vi "Parse Sentence_GGA.vi"(8 "error in (no error)":errorcluster, 11 "GGA sentence":string) -> (0 "error out":errorcluster, 3 "GGA_Data":T1 {"fix quality"."quality" items=["Invalid", "GPS Fix", "DGPS Fix", "PPS Fix", "Real Time Kinematic", "Float RTK", "Estimated", "Manual Input Mode", "Simulation Mode"]})   [LabVIEW 2024]
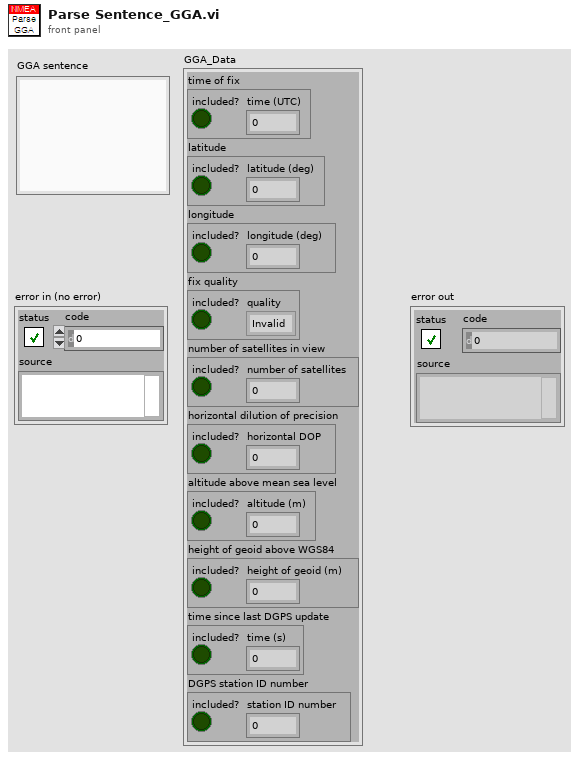
[diagram p1: front panel]
types:
  T1 = cluster{"time of fix":cluster{"included?":bool, "time (UTC)":dbl}, "latitude":cluster{"included?":bool, "latitude (deg)":dbl}, "longitude":cluster{"included?":bool, "longitude (deg)":dbl}, "fix quality":cluster{"included?":bool, "quality":u16}, "number of satellites in view":cluster{"included?":bool, "number of satellites":i8}, "horizontal dilution of precision":cluster{"included?":bool, "horizontal DOP":dbl}, "altitude above mean sea level":cluster{"included?":bool, "altitude (m)":dbl}, "height of geoid above WGS84":cluster{"included?":bool, "height of geoid (m)":dbl}, "time since last DGPS update":cluster{"included?":bool, "time (s)":dbl}, "DGPS station ID number":cluster{"included?":bool, "station ID number":dbl}}
  T2 = cluster{"Valid?":bool, "Number of Satellites":i8}
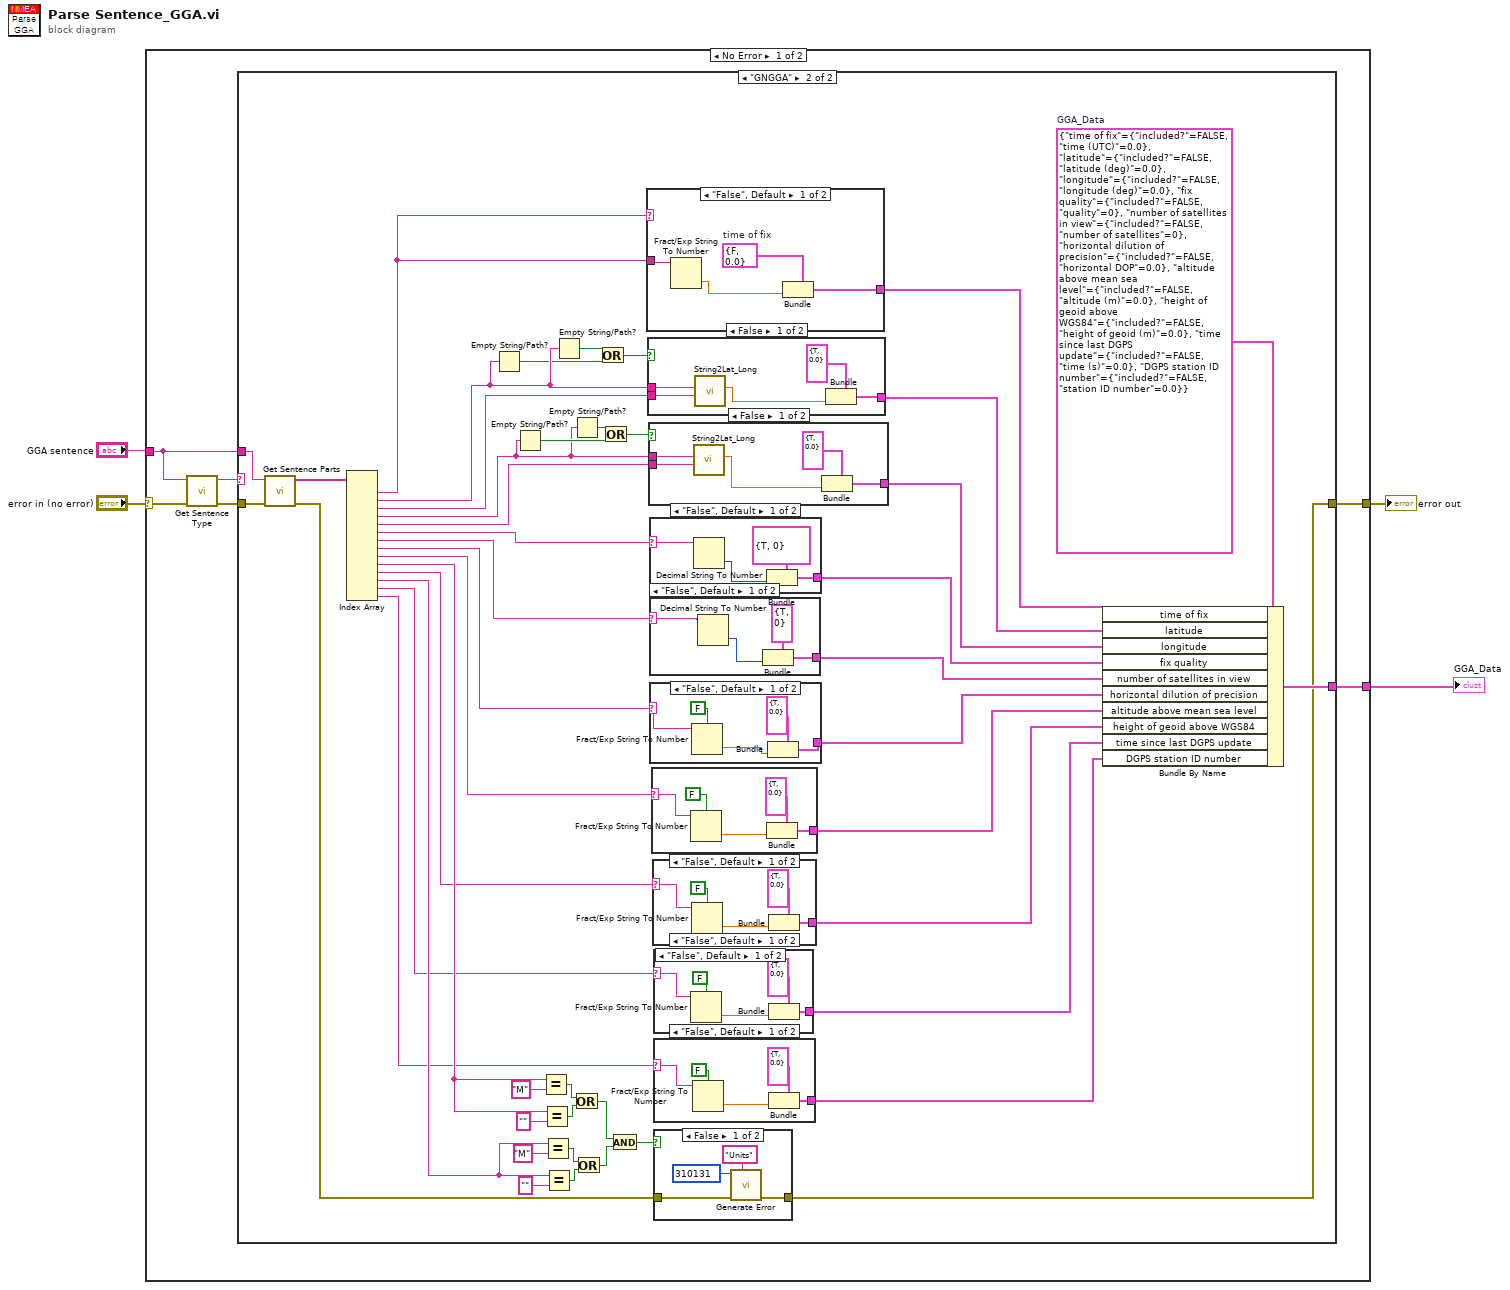
[diagram p0: block diagram]
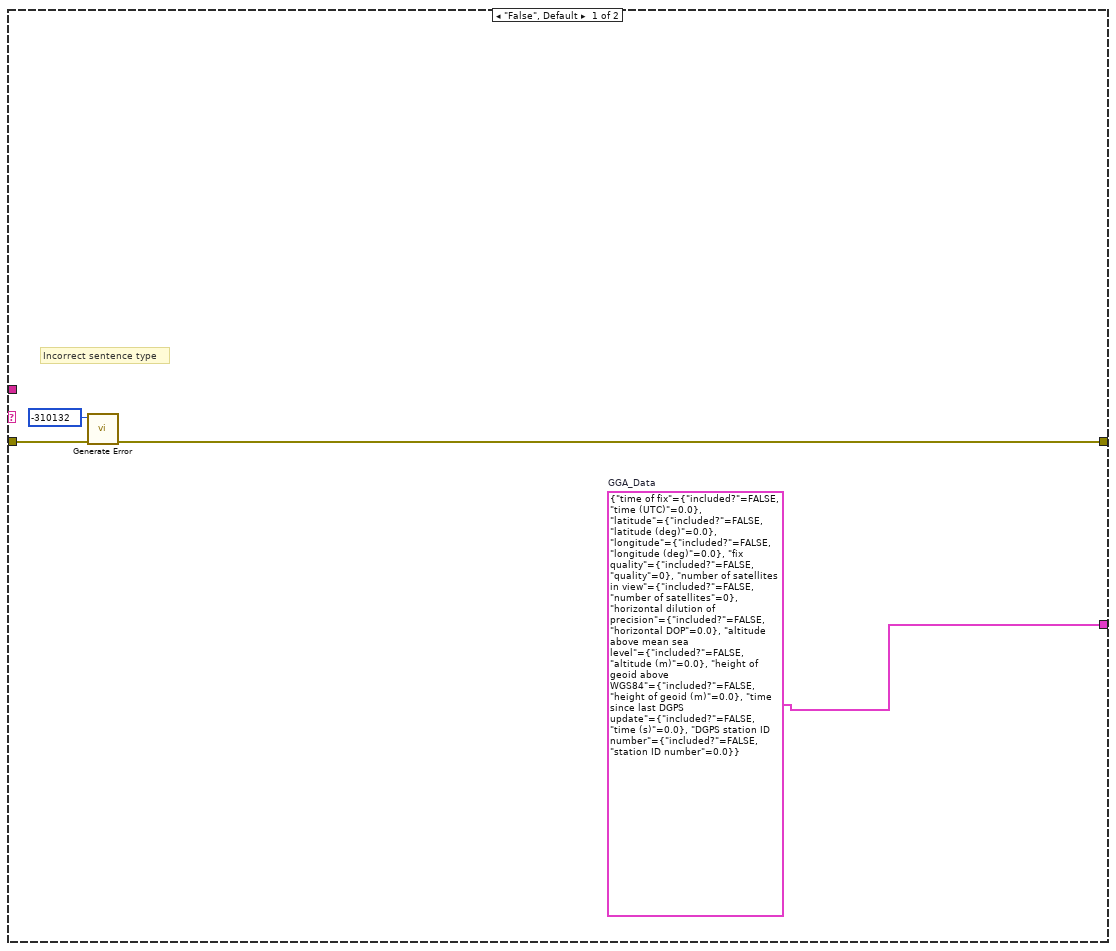
[diagram p2: hidden frame]
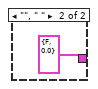
[diagram p4: hidden frame]
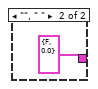
[diagram p5: hidden frame]
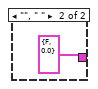
[diagram p6: hidden frame]
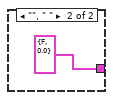
[diagram p7: hidden frame]
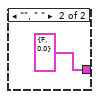
[diagram p8: hidden frame]
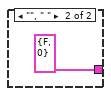
[diagram p9: hidden frame]
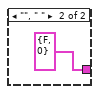
[diagram p10: hidden frame]
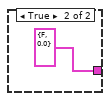
[diagram p11: hidden frame]
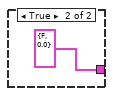
[diagram p12: hidden frame]
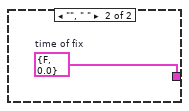
[diagram p13: hidden frame]
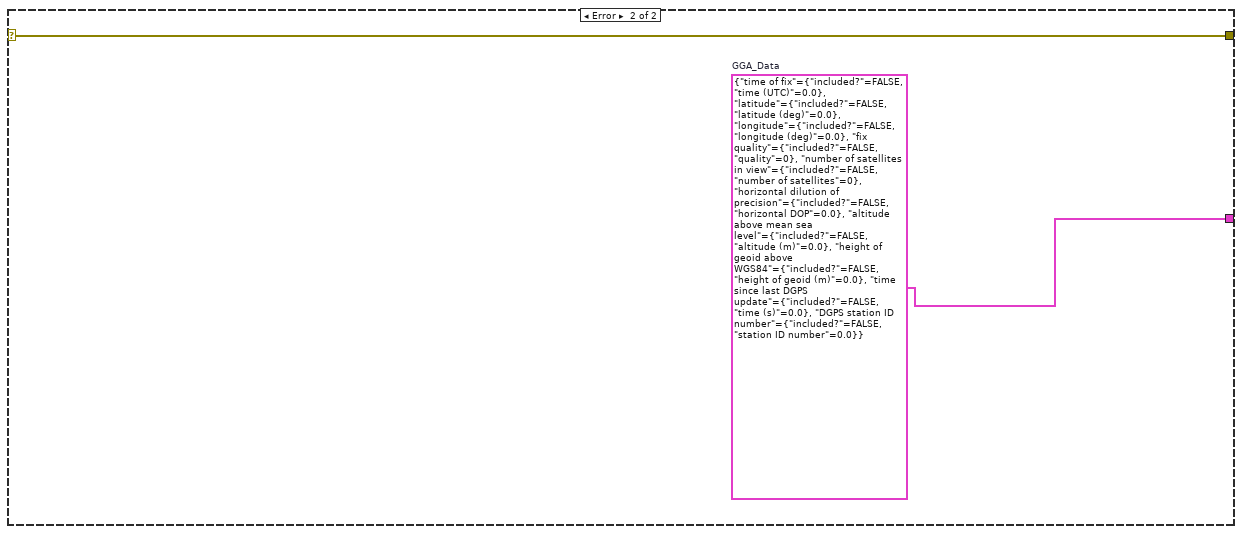
[diagram p14: hidden frame]
diagram:
  n1 = case shown="No Error" "error in (no error)" {
    selector: "error in (no error)" -> [w8 w126]
    tunnel: [w9 w126] -> w2
    tunnel: [w10 w125] -> w1
    tunnel: "GGA sentence" -> [w6 _]
    frame No Error {
      n2 = call "Get Sentence Type.vi"("error in (no error)"=w8, "sentence"=w6) -> ("error out"=w7:errorcluster, "sentence type"=w5:string)  [unwired: 7 in, 1 out]
      n3 = case shown="\"GNGGA\"" w5 {
        tunnel: [w11 w62] -> w10
        tunnel: w6 -> [_ w18]
        tunnel: w7 -> [w13 w61]
        tunnel: [w12 w42] -> w9
        frame "False", Default {
          w11 = T1 {"time of fix"={"included?"=FALSE, "time (UTC)"=0.0}, "latitude"={"included?"=FALSE, "latitude (deg)"=0.0}, "longitude"={"included?"=FALSE, "longitude (deg)"=0.0}, "fix quality"={"included?"=FALSE, "quality"=0}, "number of satellites in view"={"included?"=FALSE, "number of satellites"=0}, "horizontal dilution of precision"={"included?"=FALSE, "horizontal DOP"=0.0}, "altitude above mean sea level"={"included?"=FALSE, "altitude (m)"=0.0}, "height of geoid above WGS84"={"included?"=FALSE, "height of geoid (m)"=0.0}, "time since last DGPS update"={"included?"=FALSE, "time (s)"=0.0}, "DGPS station ID number"={"included?"=FALSE, "station ID number"=0.0}}  # GGA_Data
          # "Incorrect sentence type"
          n4 = call "Generate Error.vi"("error in (no error)"=w13, "code"=-310132) -> ("error out"=w12:errorcluster)  [unwired: 9 in]
        }
        frame "GNGGA" {
          w16 = T1 {"time of fix"={"included?"=FALSE, "time (UTC)"=0.0}, "latitude"={"included?"=FALSE, "latitude (deg)"=0.0}, "longitude"={"included?"=FALSE, "longitude (deg)"=0.0}, "fix quality"={"included?"=FALSE, "quality"=0}, "number of satellites in view"={"included?"=FALSE, "number of satellites"=0}, "horizontal dilution of precision"={"included?"=FALSE, "horizontal DOP"=0.0}, "altitude above mean sea level"={"included?"=FALSE, "altitude (m)"=0.0}, "height of geoid above WGS84"={"included?"=FALSE, "height of geoid (m)"=0.0}, "time since last DGPS update"={"included?"=FALSE, "time (s)"=0.0}, "DGPS station ID number"={"included?"=FALSE, "station ID number"=0.0}}  # GGA_Data
          n5 = call "Get Sentence Parts.vi"("error in (no error)"=w61, "sentence"=w18) -> ("error out"=w46:errorcluster, "sentence data"=w17:string[])  [unwired: 7 in, 1 out]
          n6 = Index Array(array=w17) -> (element #1=w26:string, element #2=w56:string, element #3=w60:string, element #4=w52:string, element #5=w59:string, element #6=w25:string, element #7=w24:string, element #8=w23:string, element #9=w22:string, element #10=w41:string, element #11=w21:string, element #12=w35:string, element #13=w20:string, element #14=w19:string)  [unwired: 14 in]
          n7 = Empty String/Path?(string/path=w56) -> (empty?=w55:bool)
          n8 = Empty String/Path?(string/path=w52) -> (empty?=w54:bool)
          n9 = Equal?(x=w41, y="M") -> (x = y?=w44:bool)
          n10 = Equal?(x=w41, y="") -> (x = y?=w45:bool)
          n11 = Equal?(x=w35, y="M") -> (x = y?=w37:bool)
          n12 = Equal?(x=w35, y="") -> (x = y?=w36:bool)
          n13 = Empty String/Path?(string/path=w56) -> (empty?=w57:bool)
          n14 = Empty String/Path?(string/path=w52) -> (empty?=w53:bool)
          n15 = Or(x=w44, y=w45) -> (x .or. y?=w33:bool)
          n16 = Or(x=w37, y=w36) -> (x .or. y?=w32:bool)
          n17 = Or(x=w57, y=w55) -> (x .or. y?=w58:bool)
          n18 = Or(x=w53, y=w54) -> (x .or. y?=w51:bool)
          n19 = And(x=w33, y=w32) -> (x .and. y?=w34:bool)
          n20 = case shown="\"False\", Default" w26 {
            tunnel: [w123 w124] -> w15
            tunnel: w26 -> [w121 _]
            frame "False", Default {
              w122 = cluster{"included?":bool, "time (UTC)":dbl} {"included?"=FALSE, "time (UTC)"=0.0}  # time of fix
              n21 = Fract/Exp String To Number(string=w121) -> (number=w120:dbl)  [unwired: 4 out]
              n22 = Bundle(cluster=w122, "time (UTC)"=w120) -> (w123:cluster{"included?":bool, "time (UTC)":dbl})  [unwired: 1 out]
            }
            frame "", " " {
              w124 = cluster{"included?":bool, "time (UTC)":dbl} {"included?"=FALSE, "time (UTC)"=0.0}  # time of fix
            }
          }
          n23 = case shown="False" w58 {
            tunnel: [w116 cluster{"Valid?":bool, "Latitude (Deg)":dbl} {"Valid?"=FALSE, "Latitude (Deg)"=0.0} ("Latitude")] -> w48
            tunnel: w56 -> [w118 _]
            tunnel: w60 -> [w117 _]
            frame False {
              n24 = call "String2Lat_Long.vi"("direction string"=w117, "numeric string for lat/lon"=w118) -> ("composite value"=w114:dbl)  [unwired: 9 in]
              n25 = Bundle(cluster=cluster{"Valid?":bool, "Latitude (Deg)":dbl} {"Valid?"=TRUE, "Latitude (Deg)"=0.0} ("Latitude"), "Latitude (Deg)"=w114) -> (w116:cluster{"Valid?":bool, "Latitude (Deg)":dbl})  [unwired: 1 out]
            }
            frame True {
            }
          }
          n26 = case shown="False" w51 {
            tunnel: w59 -> [w112 _]
            tunnel: w52 -> [w111 _]
            tunnel: [w108 cluster{"Valid?":bool, "Longitude (Deg)":dbl} {"Valid?"=FALSE, "Longitude (Deg)"=0.0} ("Longitude")] -> w47
            frame False {
              n27 = call "String2Lat_Long.vi"("direction string"=w112, "numeric string for lat/lon"=w111) -> ("composite value"=w110:dbl)  [unwired: 9 in]
              n28 = Bundle(cluster=cluster{"Valid?":bool, "Longitude (Deg)":dbl} {"Valid?"=TRUE, "Longitude (Deg)"=0.0} ("Longitude"), "Longitude (Deg)"=w110) -> (w108:cluster{"Valid?":bool, "Longitude (Deg)":dbl})  [unwired: 1 out]
            }
            frame True {
            }
          }
          n29 = case shown="\"False\", Default" w25 {
            selector: w25 -> [w103 _]
            tunnel: [w104 cluster{"Valid?":bool, "Fix Quality":u16} {"Valid?"=FALSE, "Fix Quality"=0} ("Fix Quality")] -> w50
            frame "False", Default {
              n30 = Decimal String To Number(string=w103) -> (number=w105:i32)  [unwired: 3 out]
              n31 = Bundle(cluster=cluster{"Valid?":bool, "Fix Quality":u16} {"Valid?"=TRUE, "Fix Quality"=0} ("Fix Quality"), "Fix Quality"=w105) -> (w104:cluster{"Valid?":bool, "Fix Quality":u16})  [unwired: 1 out]
            }
            frame "", " " {
            }
          }
          n32 = case shown="\"False\", Default" w24 {
            selector: w24 -> [w98 _]
            tunnel: [w99 T2 {"Valid?"=FALSE, "Number of Satellites"=0} ("Number of Satellites Being Tracked")] -> w49
            frame "False", Default {
              n33 = Decimal String To Number(string=w98) -> (number=w101:i32)  [unwired: 3 out]
              n34 = Bundle(cluster=T2 {"Valid?"=TRUE, "Number of Satellites"=0} ("Number of Satellites Being Tracked"), "Number of Satellites"=w101) -> (w99:T2)  [unwired: 1 out]
            }
            frame "", " " {
            }
          }
          n35 = case shown="\"False\", Default" w23 {
            selector: w23 -> [w93 _]
            tunnel: [w94 cluster{"Valid?":bool, "Horizontal DOP":dbl} {"Valid?"=FALSE, "Horizontal DOP"=0.0} ("Horizontal Dilution of Precision")] -> w31
            frame "False", Default {
              n36 = Fract/Exp String To Number(use system decimal point (T)=FALSE, string=w93) -> (number=w95:dbl)  [unwired: 3 out]
              n37 = Bundle(cluster=cluster{"Valid?":bool, "Horizontal DOP":dbl} {"Valid?"=TRUE, "Horizontal DOP"=0.0} ("Horizontal Dilution of Precision"), "Horizontal DOP"=w95) -> (w94:cluster{"Valid?":bool, "Horizontal DOP":dbl})  [unwired: 1 out]
            }
            frame "", " " {
            }
          }
          n38 = case shown="\"False\", Default" w22 {
            selector: w22 -> [w87 _]
            tunnel: [w88 cluster{"Valid?":bool, "Horizontal DOP":dbl} {"Valid?"=FALSE, "Horizontal DOP"=0.0} ("Horizontal Dilution of Precision")] -> w30
            frame "False", Default {
              n39 = Fract/Exp String To Number(use system decimal point (T)=FALSE, string=w87) -> (number=w89:dbl)  [unwired: 3 out]
              n40 = Bundle(cluster=cluster{"Valid?":bool, "Horizontal DOP":dbl} {"Valid?"=TRUE, "Horizontal DOP"=0.0} ("Horizontal Dilution of Precision"), "Horizontal DOP"=w89) -> (w88:cluster{"Valid?":bool, "Horizontal DOP":dbl})  [unwired: 1 out]
            }
            frame "", " " {
            }
          }
          n41 = case shown="\"False\", Default" w21 {
            selector: w21 -> [w81 _]
            tunnel: [w82 cluster{"Valid?":bool, "Horizontal DOP":dbl} {"Valid?"=FALSE, "Horizontal DOP"=0.0} ("Horizontal Dilution of Precision")] -> w29
            frame "False", Default {
              n42 = Fract/Exp String To Number(use system decimal point (T)=FALSE, string=w81) -> (number=w83:dbl)  [unwired: 3 out]
              n43 = Bundle(cluster=cluster{"Valid?":bool, "Horizontal DOP":dbl} {"Valid?"=TRUE, "Horizontal DOP"=0.0} ("Horizontal Dilution of Precision"), "Horizontal DOP"=w83) -> (w82:cluster{"Valid?":bool, "Horizontal DOP":dbl})  [unwired: 1 out]
            }
            frame "", " " {
            }
          }
          n44 = case shown="\"False\", Default" w20 {
            selector: w20 -> [w75 _]
            tunnel: [w76 cluster{"Valid?":bool, "Horizontal DOP":dbl} {"Valid?"=FALSE, "Horizontal DOP"=0.0} ("Horizontal Dilution of Precision")] -> w28
            frame "False", Default {
              n45 = Fract/Exp String To Number(use system decimal point (T)=FALSE, string=w75) -> (number=w77:dbl)  [unwired: 3 out]
              n46 = Bundle(cluster=cluster{"Valid?":bool, "Horizontal DOP":dbl} {"Valid?"=TRUE, "Horizontal DOP"=0.0} ("Horizontal Dilution of Precision"), "Horizontal DOP"=w77) -> (w76:cluster{"Valid?":bool, "Horizontal DOP":dbl})  [unwired: 1 out]
            }
            frame "", " " {
            }
          }
          n47 = case shown="\"False\", Default" w19 {
            selector: w19 -> [w69 _]
            tunnel: [w70 cluster{"Valid?":bool, "Horizontal DOP":dbl} {"Valid?"=FALSE, "Horizontal DOP"=0.0} ("Horizontal Dilution of Precision")] -> w27
            frame "False", Default {
              n48 = Fract/Exp String To Number(use system decimal point (T)=FALSE, string=w69) -> (number=w71:dbl)  [unwired: 3 out]
              n49 = Bundle(cluster=cluster{"Valid?":bool, "Horizontal DOP":dbl} {"Valid?"=TRUE, "Horizontal DOP"=0.0} ("Horizontal Dilution of Precision"), "Horizontal DOP"=w71) -> (w70:cluster{"Valid?":bool, "Horizontal DOP":dbl})  [unwired: 1 out]
            }
            frame "", " " {
            }
          }
          n50 = case shown="False" w34 {
            tunnel: w46 -> [w65 w67]
            tunnel: [w64 w67] -> w42
            frame False {
              n51 = call "Generate Error.vi"("<append> (\"\")"="Units" ("<append> (\"\")"), "error in (no error)"=w65, "code"=310131) -> ("error out"=w64:errorcluster)  [unwired: 8 in]
            }
            frame True {
            }
          }
          n52 = Bundle By Name(cluster=w16, "time of fix"=w15, "latitude"=w48, "longitude"=w47, "fix quality"=w50, "number of satellites in view"=w49, "horizontal dilution of precision"=w31, "altitude above mean sea level"=w30, "height of geoid above WGS84"=w29, "time since last DGPS update"=w28, "DGPS station ID number"=w27) -> (w62:T1)
        }
      }
    }
    frame Error {
      w125 = T1 {"time of fix"={"included?"=FALSE, "time (UTC)"=0.0}, "latitude"={"included?"=FALSE, "latitude (deg)"=0.0}, "longitude"={"included?"=FALSE, "longitude (deg)"=0.0}, "fix quality"={"included?"=FALSE, "quality"=0}, "number of satellites in view"={"included?"=FALSE, "number of satellites"=0}, "horizontal dilution of precision"={"included?"=FALSE, "horizontal DOP"=0.0}, "altitude above mean sea level"={"included?"=FALSE, "altitude (m)"=0.0}, "height of geoid above WGS84"={"included?"=FALSE, "height of geoid (m)"=0.0}, "time since last DGPS update"={"included?"=FALSE, "time (s)"=0.0}, "DGPS station ID number"={"included?"=FALSE, "station ID number"=0.0}}  # GGA_Data
    }
  }
  "error out" <- w2
  "GGA_Data" <- w1
